vi "Format GroupItemType_LVXML_GroupSet.vi"(8 "error in (no error)":errorcluster, 10 "valueXmlData":T2, 11 "AWS_EC2 in":refnum<class "AWS_EC2.lvclass">) -> (0 "error out":errorcluster, 2 "Array":T3[](array[typedef]), 3 "AWS_EC2 out":refnum<class "AWS_EC2.lvclass">)   [LabVIEW 2014, in "AWS_EC2.lvlib" / "AWS_EC2.lvclass"]
uses:
  AWS_EC2.lvclass
  lv-xml-parser/r0/trunk/VI Source/LV XML Parser.lvlib
  EC2 Datatypes/GroupItemType.ctl
  AWS_EC2.lvlib
  lv-xml-parser/r0/trunk/VI Source/EventType.ctl
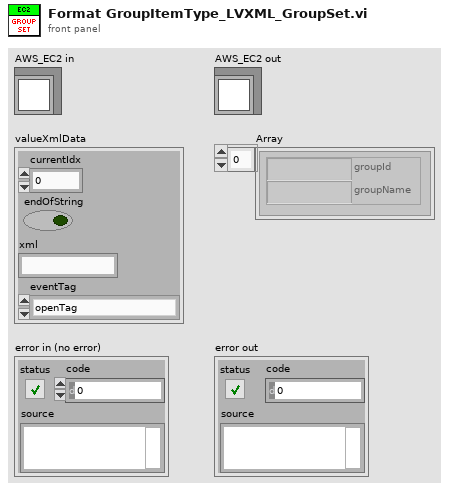
[diagram p1: front panel]
types:
  T1 = typedef "LV XML Parser.lvlib/EventType.ctl" = enum16{"openTag", "endOpenTag", "closeTag", "comment", "endComment", "endOfFile", "attribute", "startXml"}
  T2 = cluster{"currentIdx":i32, "endOfString":bool, "xml":string, "eventTag":T1}
  T3 = typedef "AWS_EC2.lvlib/GroupItemType.ctl" = cluster{"groupId":string, "groupName":string}
  T4 = cluster{"namespaceUri":string, "localName":string}
  T5 = cluster{"Attributes":cluster{"localName":string, "namespaceUri":string, "value":string}[], "localName":string, "namespaceUri":string, "valueXmlData":cluster{"currentIdx":i32, "endOfString":bool, "xml":string, "eventTag":T1}}[]
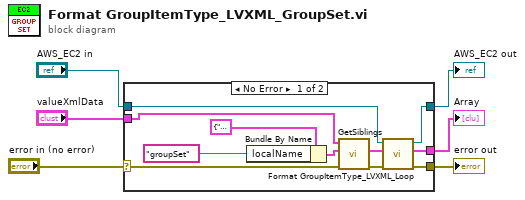
[diagram p0: block diagram]
diagram:
  n1 = case shown="No Error" "error in (no error)" {
    selector: "error in (no error)" -> [w13 w18]
    tunnel: [w8 w19] -> w2
    tunnel: "AWS_EC2 in" -> [w7 w19]
    tunnel: [w12 w18] -> w4
    tunnel: "valueXmlData" -> [w17 _]
    tunnel: [w9 _] -> w6
    frame No Error {
      n2 = Bundle By Name(cluster=T4 {"namespaceUri"="", "localName"=""} ("limitToTag"), "localName"="groupSet" ("Tag name")) -> (w14:T4)
      n3 = call "GetSiblings.vi"("error in (no error)"=w13, "limitToTag"=w14, "xmlData"=w17) -> ("error out"=w11:errorcluster, "Siblings"=w10:T5)  [unwired: 7 in]
      n4 = call "Format GroupItemType_LVXML_Loop.vi"("error in (no error)"=w11, "Siblings in"=w10, "AWS_EC2 in"=w7) -> ("error out"=w12:errorcluster, "Array"=w9:T3[], "AWS_EC2 out"=w8:refnum<class "AWS_EC2.lvclass">)  [unwired: 6 in]
    }
    frame Error {
    }
  }
  "Array" <- w6
  "error out" <- w4
  "AWS_EC2 out" <- w2
